vi "ReadHEKA.vi"(8 "Error IN":errorcluster, 9 "Mode?":enum16{"V-mode", "C-mode"}(ring), 11 "FilePath":path) -> (0 "Error OUT":errorcluster, 1 "File Parameters":T1, 3 "Traces":sgl[][](array[numeric]))   [LabVIEW 2017]
uses:
  HEKAdat.lvclass
  File Parameters.ctl
panel:
  in  "HEKAdat.lvclass IN":refnum<class "HEKAdat.lvclass">
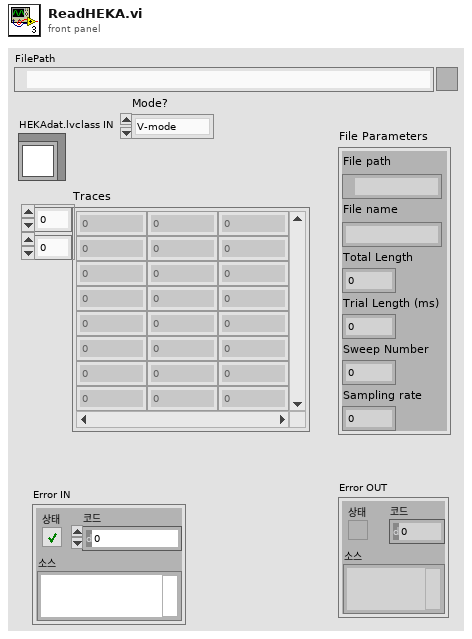
[diagram p1: front panel]
types:
  T1 = typedef "File Parameters.ctl" = cluster{"File path":path, "File name":string, "Total Length":i32, "Trial Length (ms)":i32, "Sweep Number":i32, "Sampling rate":dbl}
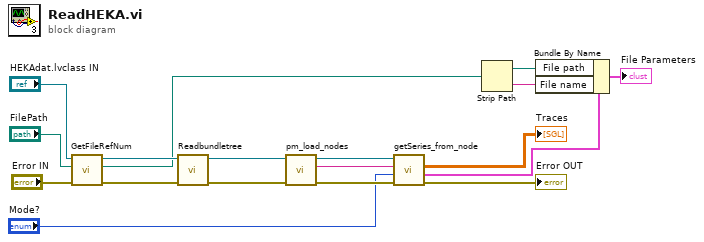
[diagram p0: block diagram]
diagram:
  n1 = call "GetFileRefNum.vi"("Error IN"="Error IN", "FilePath"="FilePath", "HEKAdat.lvclass IN"="HEKAdat.lvclass IN") -> ("Error OUT"=w17:errorcluster, "FilePath"=w9:path, "HEKAdat.lvclass OUT"=w18:refnum<class "HEKAdat.lvclass">)  [unwired: 6 in]
  n2 = call "Readbundletree.vi"("Error IN"=w17, "HEKAdat.lvclass IN"=w18) -> ("Error OUT"=w15:errorcluster, "HEKAdat.lvclass OUT"=w14:refnum<class "HEKAdat.lvclass">)  [unwired: 8 in]
  n3 = call "pm_load_nodes.vi"("Error IN"=w15, "HEKAdat.lvclass IN"=w14) -> ("Error OUT"=w12:errorcluster, "Selected item"=w10:string, "HEKAdat.lvclass OUT"=w13:refnum<class "HEKAdat.lvclass">)  [unwired: 7 in]
  n4 = call "getSeries_from_node.vi"("Error IN"=w12, "Mode?"="Mode?", "Selected item"=w10, "HEKAdat.lvclass IN"=w13) -> ("Error OUT"=→"Error OUT":errorcluster, "File Parameters OUT"=w6:T1, "Traces"=→"Traces":sgl[][])  [unwired: 4 in, 1 out]
  n5 = Strip Path(path=w9) -> (stripped path=w8:path, name=w7:string)
  n6 = Bundle By Name(cluster=w6, "File path"=w8, "File name"=w7) -> (→"File Parameters":T1)
